vi "UDP_read.vi"() -> ()   [LabVIEW 2010]
panel:
  in  "error in":errorcluster
  out "Temperature":dbl=52.16291 format="%.2f"
  out "String":string="52.162910\r\n"
  out "error out":errorcluster
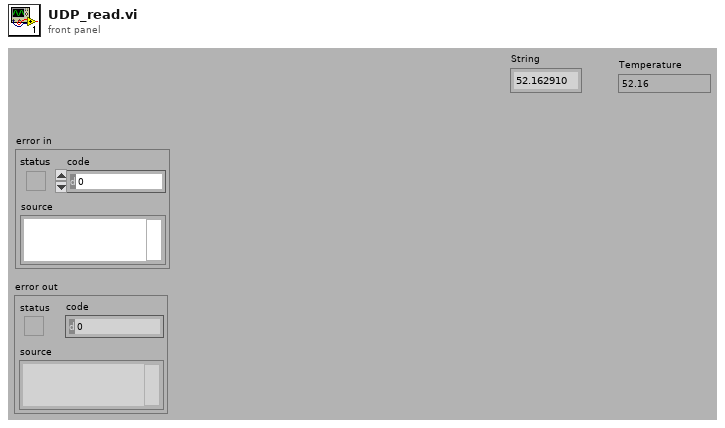
[diagram p1: front panel]
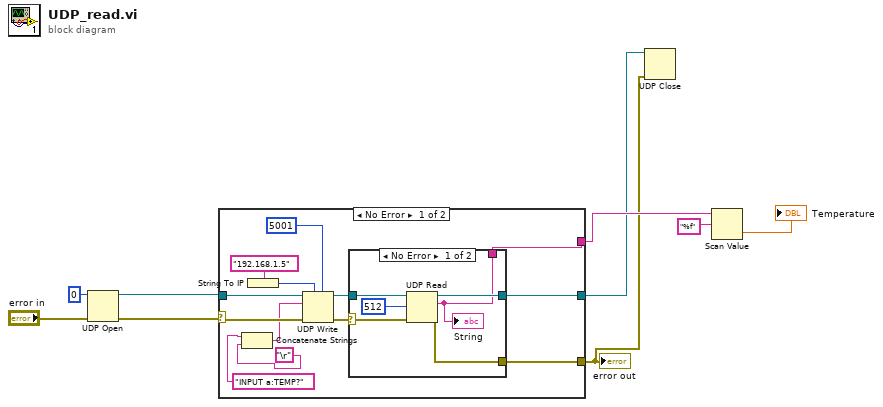
[diagram p0: block diagram]
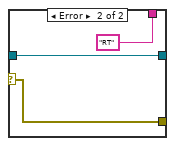
[diagram p2: hidden frame]
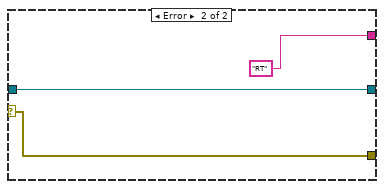
[diagram p3: hidden frame]
diagram:
  n1 = UDP Open(8:"error in", 11:0) -> (port=w4:refnum<k16>, 0:w3:errorcluster)  [unwired: 3 in, 1 out]
  n2 = case shown="No Error" w3 {
    selector: w3 -> [w22 w34]
    tunnel: [w18 w34] -> w1
    tunnel: w4 -> [w21 w32]
    tunnel: [w12 "RT" ("Sub folder")] -> w5
    tunnel: [w11 w32] -> w2
    frame No Error {
      n3 = Concatenate Strings("INPUT a:TEMP?", "\r") -> (w13:string)
      n4 = String To IP(1:"192.168.1.5") -> (0:w15:u32)
      n5 = UDP Write(address=w15, port or service name=u16 5001, connection ID=w21, data in=w13, 8:w22) -> (error out=w20:errorcluster, 3:w19:refnum<k16>)  [unwired: 1 in]
      n6 = case shown="No Error" w20 {
        selector: w20 -> [w28 w30]
        tunnel: w19 -> [w27 w31]
        tunnel: [w25 w31] -> w11
        tunnel: [w24 w30] -> w18
        tunnel: [w23 "RT" ("Sub folder")] -> w12
        frame No Error {
          n7 = UDP Read(connection ID=w27, max size (548)=512, 8:w28) -> (data out=w23:string, error out=w24:errorcluster, 3:w25:refnum<k16>)  [unwired: 1 in, 2 out]
          "String" <- w23
        }
        frame Error {
        }
      }
    }
    frame Error {
    }
  }
  "error out" <- w1
  n8 = UDP Close(connection ID=w2, 8:w1) -> ()  [unwired: 2 out]
  n9 = Scan Value(string=w5, format string="%f") -> (value=→"Temperature":dbl)  [unwired: 1 in, 1 out]
